vi "Functional Imaging-Extract ROI overlay info.vi"(9 "Functional Imging UI Refs":T4, 10 "Functional Parameters":T6, 11 "[ROI]":T1 caption="[POI]" {"ROI number" min=1 format="ROI %.0f"}) -> (1 "[ROI index] (unity based)":i32[](array[numeric]), 3 "[ROI info]":T7[](array[typedef]) {"Apparent Frame Size" format="%#_6f"; "Original FOV (um)" format="%#_6f"; "Pixels per miniscan" format="%#_6f"; "Dwell Time per pixel" format="%#_6f"; "Resolution" format="%#_6f"; "ROI group ID" format="%#_6f"; "Laser Power (%)" format="%#_6f"; "Zoom" format="%#_6f"; "Frame Size" format="%#_6f"; "Number of lines" format="%#_6f"; "Composite ID" format="%#_6f"; "Angle (deg)" format="%#_6f"; "ROI Time (ns)" format="%#_6f"; "ROI ID" format="%#_6f"; "Pixels in ROI" format="%#_6f"; "ROI index" format="%#_6f"; "Z stop" format="%#_6f"; "Y stop" format="%#_6f"; "X stop" format="%#_6f"; "Z start" format="%#_6f"; "X start" format="%#_6f"; "Y start" format="%#_6f"})   [LabVIEW 2020]
uses:
  Typedefs/ROI parameters data type.ctl
  Typedefs/Functional Parameters Cluster.ctl
  Typedefs/Functional Imging UI Refs.ctl
  xcontrol/XGrapher.xctl
  Typedefs/ROI selector array-ROI vis.ctl
  xcontrol/Interface VIs/Interface typedefs/Interface-ROI selection cluster.ctl
  Typedefs/ROI ID Enum.ctl
  Typedefs/Groups array referecne.ctl
  Typedefs/ROI visibility mode.ctl
panel:
  # "[Groups] is a Typedef"
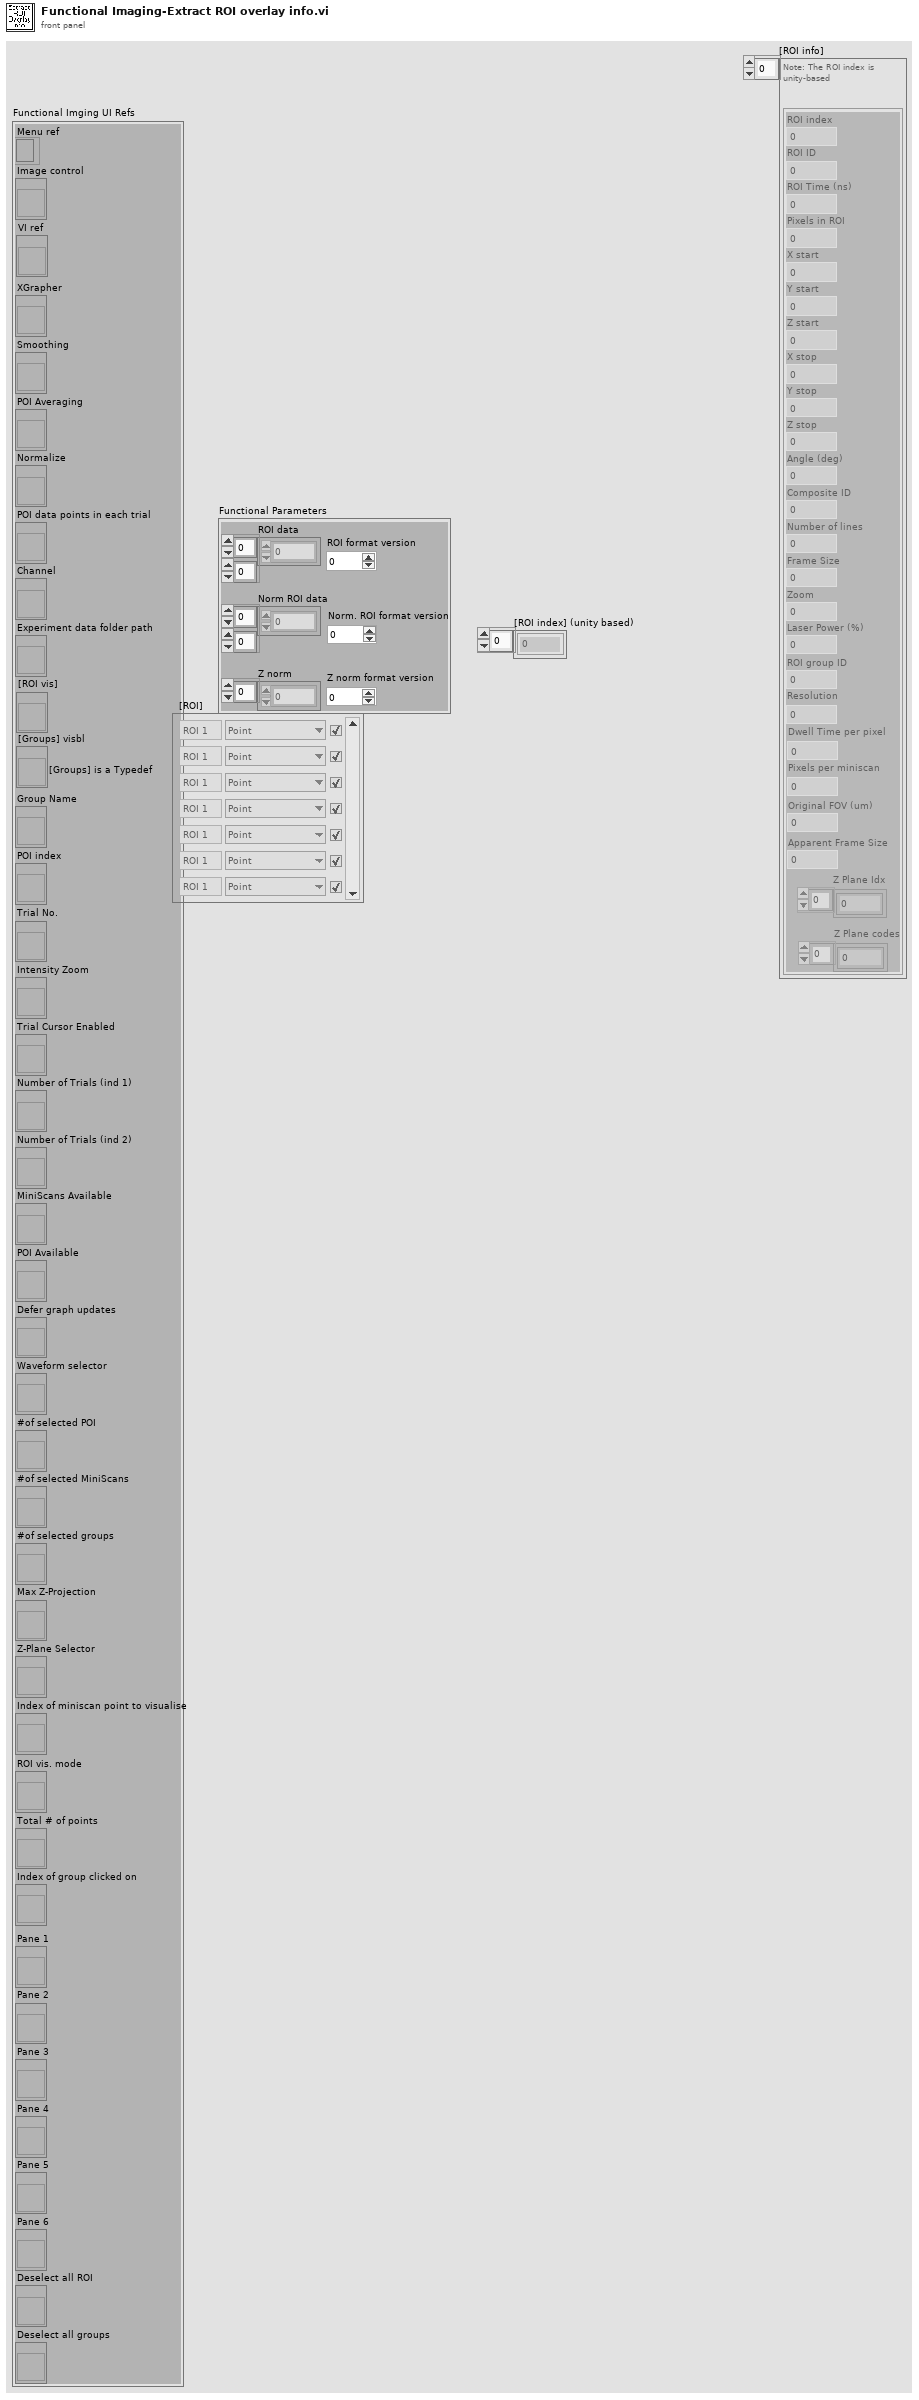
[diagram p1: front panel]
types:
  T1 = typedef "ROI selector array-ROI vis.ctl" = T2[]
  T2 = typedef "Interface-ROI selection cluster.ctl" = cluster{"ROI number":i32, "ROI ID":T3, "Visibility":bool}
  T3 = typedef "ROI ID Enum.ctl" = enum16{"Point", "MiniScan", "Comp. MiniScan", "Rectangle", "Comp. volume", "Arb. plane point", "None"}
  T4 = typedef "Functional Imging UI Refs.ctl" = cluster{"Menu ref":refnum<k9>, "Image control":refnum<vi>, "VI ref":refnum<vi>, "XGrapher":refnum<vi>, "Smoothing":refnum<vi>, "POI Averaging":refnum<vi>, "Normalize":refnum<vi>, "POI data points in each trial":refnum<vi>, "Channel":refnum<vi>, "Experiment data folder path":refnum<vi>, "[ROI vis]":refnum<vi>, "[Groups] visbl":T5, "Group Name":refnum<vi>, "POI index":refnum<vi>, "Trial No.":refnum<vi>, "Intensity Zoom":refnum<vi>, "Trial Cursor Enabled":refnum<vi>, "Number of Trials (ind 1)":refnum<vi>, "Number of Trials (ind 2)":refnum<vi>, "MiniScans Available":refnum<vi>, "POI Available":refnum<vi>, "Defer graph updates":refnum<vi>, "Waveform selector":refnum<vi>, "#of selected POI":refnum<vi>, "#of selected MiniScans":refnum<vi>, "#of selected groups":refnum<vi>, "Max Z-Projection":refnum<vi>, "Z-Plane Selector":refnum<vi>, "Index of miniscan point to visualise":refnum<vi>, "ROI vis. mode":refnum<vi>, "Total # of points":refnum<vi>, "Index of group clicked on":refnum<vi>, "Pane 1":refnum<vi>, "Pane 2":refnum<vi>, "Pane 3":refnum<vi>, "Pane 4":refnum<vi>, "Pane 5":refnum<vi>, "Pane 6":refnum<vi>, "Deselect all ROI":refnum<vi>, "Deselect all groups":refnum<vi>}
  T5 = typedef "Groups array referecne.ctl" = refnum<vi>
  T6 = typedef "Functional Parameters Cluster.ctl" = cluster{"ROI data":dbl[][], "ROI format version":i32, "Norm ROI data":dbl[][], "Norm. ROI format version":i32, "Z norm":dbl[], "Z norm format version":i32}
  T7 = typedef "ROI parameters data type.ctl" = cluster{"ROI index":dbl, "ROI ID":dbl, "ROI Time (ns)":dbl, "Pixels in ROI":dbl, "X start":dbl, "Y start":dbl, "Z start":dbl, "X stop":dbl, "Y stop":dbl, "Z stop":dbl, "Angle (deg)":dbl, "Composite ID":dbl, "Number of lines":dbl, "Frame Size":dbl, "Zoom":dbl, "Laser Power (%)":dbl, "ROI group ID":dbl, "Resolution":dbl, "Dwell Time per pixel":dbl, "Pixels per miniscan":dbl, "Original FOV (um)":dbl, "Apparent Frame Size":dbl, "Z Plane Idx":i32[], "Z Plane codes":i32[]}
  T8 = typedef "ROI visibility mode.ctl" = enum16{"Show all ROI when scrolling in Z", "Show only selected ROI when scrolling in Z"}
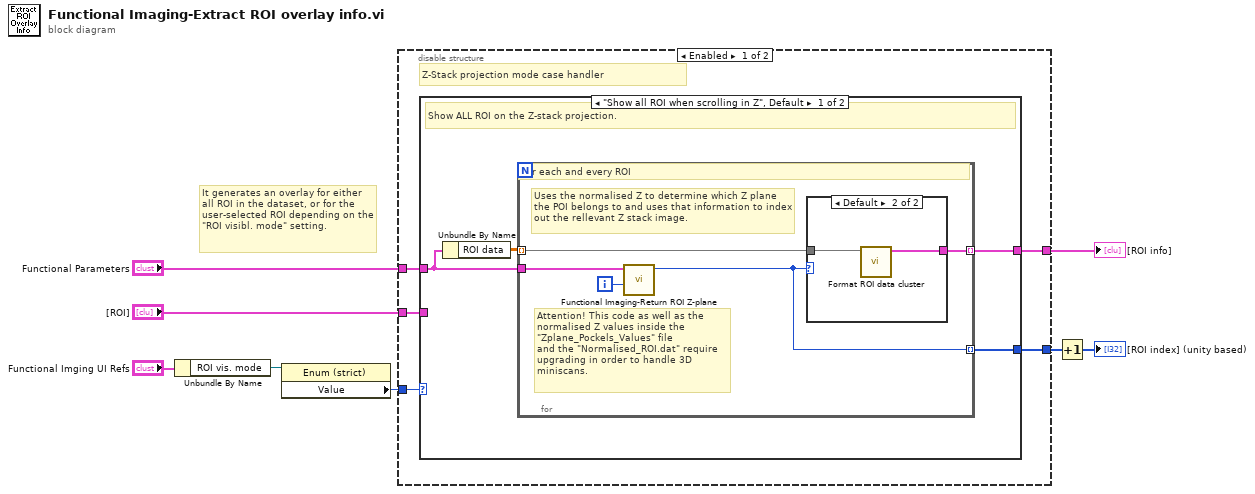
[diagram p0: block diagram]
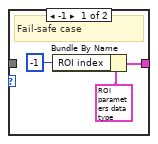
[diagram p2: hidden frame]
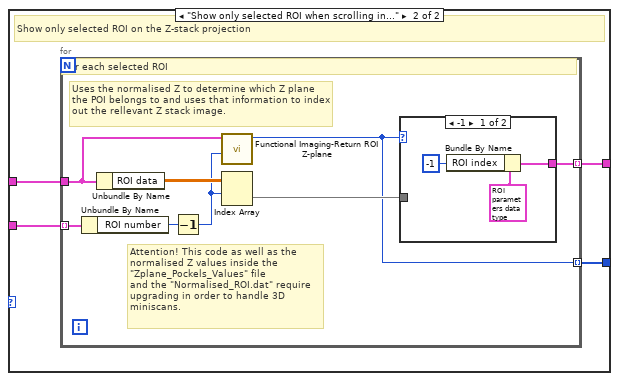
[diagram p3: hidden frame]
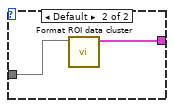
[diagram p4: hidden frame]
diagram:
  # "It generates an overlay for either all ROI in the dataset, or for the user-selected ROI depending on the \"ROI visibl. mode\" setting."
  n1 = Unbundle By Name("Functional Imging UI Refs") -> ("ROI vis. mode"=w6:refnum<vi>)
  n2 = property on="Property Node" class="Enum (strict)"(reference=w6) -> ("Value"=w4:T8)  [unwired: 1 in, 2 out]
  n3 = disable-structure shown="Enabled" {
    disable-tunnel: [w13 _] -> w8
    disable-tunnel: "Functional Parameters" -> [w12 _]
    disable-tunnel: w4 -> [w11 _]
    disable-tunnel: "[ROI]" -> [w10 _]
    disable-tunnel: [w9 _] -> w1
    frame Enabled {
      # "Z-Stack projection mode case handler"
      n4 = case shown="\"Show all ROI when scrolling in Z\", Default" w11 {
        tunnel: [w17 w28] -> w13
        tunnel: [w14 w29] -> w9
        tunnel: w12 -> [w16 w30]
        tunnel: w10 -> [_ w31]
        frame "Show all ROI when scrolling in Z", Default {
          # "Show ALL ROI on the Z-stack projection."
          n5 = Unbundle By Name(w16) -> ("ROI data"=w15:dbl[][])
          n6 = for {
            tunnel: [w22] -> w17 mode=indexing
            tunnel: w15 -> [w21] mode=indexing
            tunnel: w16 -> [w20]
            tunnel: [w18] -> w14 mode=indexing
            i -> [w19]
            # "Attention! This code as well as the normalised Z values inside the \"Zplane_Pockels_Values\" file\nand the \"Normalised_ROI.dat\" require upgrading in order to handle 3D miniscans."
            # "Uses the normalised Z to determine which Z plane the POI belongs to and uses that information to index out the rellevant Z stack image."
            # "For each and every ROI"
            n7 = call "Functional Imaging-Return ROI Z-plane.vi"("ROI index (zero based)"=w19, "Functional Parameters"=w20) -> ("Zero-based index of the Z-plane the indexed ROI belongs to"=w18:i32)  [unwired: 9 in]
            n8 = case shown="Default" w18 {
              tunnel: w21 -> [_ w27]
              tunnel: [w23 w26] -> w22
              frame -1 {
                # "Fail-safe case"
                n9 = Bundle By Name(cluster=T7 {"ROI index"=0.0, "ROI ID"=0.0, "ROI Time (ns)"=0.0, "Pixels in ROI"=0.0, "X start"=0.0, "Y start"=0.0, "Z start"=0.0, "X stop"=0.0, "Y stop"=0.0, "Z stop"=0.0, "Angle (deg)"=0.0, "Composite ID"=0.0, "Number of lines"=0.0, "Frame Size"=0.0, "Zoom"=0.0, "Laser Power (%)"=0.0, "ROI group ID"=0.0, "Resolution"=0.0, "Dwell Time per pixel"=0.0, "Pixels per miniscan"=0.0, "Original FOV (um)"=0.0, "Apparent Frame Size"=0.0, "Z Plane Idx"=[], "Z Plane codes"=[]} ("X-Y-Z coordinates"), "ROI index"=i64 -1) -> (w23:T7)
              }
              frame Default {
                n10 = call "Format ROI data cluster.vi"("Single ROI info"=w27) -> ("X-Y-Z coordinates"=w26:T7)  [unwired: 10 in]
              }
            }
          }
        }
        frame "Show only selected ROI when scrolling in Z" {
          # "Show only selected ROI on the Z-stack projection"
          n11 = for {
            tunnel: w31 -> [w39] mode=indexing
            tunnel: [w37] -> w28 mode=indexing
            tunnel: w30 -> [w34]
            tunnel: [w33] -> w29 mode=indexing
            # "Attention! This code as well as the normalised Z values inside the \"Zplane_Pockels_Values\" file\nand the \"Normalised_ROI.dat\" require upgrading in order to handle 3D miniscans."
            # "Uses the normalised Z to determine which Z plane the POI belongs to and uses that information to index out the rellevant Z stack image."
            # "For each selected ROI"
            n12 = Unbundle By Name(w39) -> ("ROI number"=w35:i32)
            n13 = Unbundle By Name(w34) -> ("ROI data"=w36:dbl[][])
            n14 = Decrement(x=w35) -> (x-1=w32:i32)
            n15 = call "Functional Imaging-Return ROI Z-plane.vi"("ROI index (zero based)"=w32, "Functional Parameters"=w34) -> ("Zero-based index of the Z-plane the indexed ROI belongs to"=w33:i32)  [unwired: 9 in]
            n16 = Index Array(array=w36, index (row)=w32) -> (element=w38:dbl[])  [unwired: 1 in]
            n17 = case shown="-1" w33 {
              tunnel: w38 -> [_ w43]
              tunnel: [w40 w44] -> w37
              frame -1 {
                n18 = Bundle By Name(cluster=T7 {"ROI index"=0.0, "ROI ID"=0.0, "ROI Time (ns)"=0.0, "Pixels in ROI"=0.0, "X start"=0.0, "Y start"=0.0, "Z start"=0.0, "X stop"=0.0, "Y stop"=0.0, "Z stop"=0.0, "Angle (deg)"=0.0, "Composite ID"=0.0, "Number of lines"=0.0, "Frame Size"=0.0, "Zoom"=0.0, "Laser Power (%)"=0.0, "ROI group ID"=0.0, "Resolution"=0.0, "Dwell Time per pixel"=0.0, "Pixels per miniscan"=0.0, "Original FOV (um)"=0.0, "Apparent Frame Size"=0.0, "Z Plane Idx"=[], "Z Plane codes"=[]} ("X-Y-Z coordinates"), "ROI index"=i64 -1) -> (w40:T7)
              }
              frame Default {
                n19 = call "Format ROI data cluster.vi"("Single ROI info"=w43) -> ("X-Y-Z coordinates"=w44:T7)  [unwired: 10 in]
              }
            }
          }
        }
      }
    }
    frame Disabled {
    }
  }
  "[ROI info]" <- w8
  n20 = Increment(x=w1) -> (x+1=→"[ROI index] (unity based)":i32[])
